vi "FileExists.vi"(11 "NAS path":path) -> (3 "created path":path, 5 "Exists?":bool)   [LabVIEW 2018]
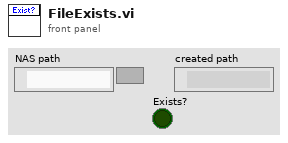
[diagram p1: front panel]
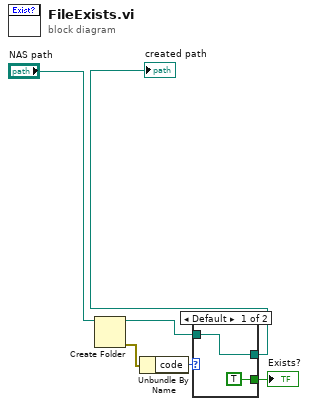
[diagram p0: block diagram]
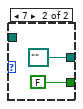
[diagram p2: hidden frame]
diagram:
  n1 = Create Folder(path (use dialog)="NAS path") -> (created path=w4:path, error out=w2:errorcluster)  [unwired: 2 in, 1 out]
  n2 = Unbundle By Name(w2) -> ("code"=w3:i32)
  n3 = case shown="Default" w3 {
    tunnel: [w8 path "" ("created path")] -> w6
    tunnel: w4 -> [w8 _]
    tunnel: [TRUE FALSE] -> w1
    frame Default {
    }
    frame 7 {
    }
  }
  "created path" <- w6
  "Exists?" <- w1
